vi "Launcher.vi"(9 "launcher_name":string, 10 "pid":u32) -> ()   [LabVIEW 2021, in "CIFLauncher.lvclass"]
uses:
  CIFLauncher.lvclass
  CIFLauncher.lvclass/CIFLauncher.ctl
  <vilib>/gRPC/LabVIEW gRPC Servicer/Servicer/Servicer.lvclass
  CIFUtilities/CIFLogs/CIFLogs.lvlib
  gRPC/CIF_Launcher_server/RPC Service/Launcher/Launcher.lvclass
  gRPC/CIF_Launcher_server/RPC Messages/cif_common_Empty.ctl
  gRPC/CIF_Launcher_server/CIF_Launcher_server.lvlib
  gRPC/CIF_Launcher_server/RPC Messages/cif_common_Version.ctl
  gRPC/CIF_Launcher_server/RPC Messages/cif_manager_PluginMetadata.ctl
  gRPC/CIF_Launcher_server/RPC Messages/cif_launcher_DiscoveredPlugin.ctl
  gRPC/CIF_Launcher_server/RPC Messages/cif_common_Status.ctl
  gRPC/CIF_Launcher_server/RPC Messages/cif_manager_LauncherType.ctl
  gRPC/CIF_Launcher_server/RPC Messages/cif_manager_LauncherInfo.ctl
  gRPC/CIF_Launcher_server/RPC Messages/cif_manager_LauncherStatus.ctl
  CIFUtilities/CIFConfigurationFile/typedef/Location Type.ctl
  CIFUtilities/CIFConfigurationFile/CIF Configuration File.lvlib
  <vilib>/Utility/LVLibp/NI_PackedLibraryUtility.lvlib
  CIFPluginManager/gRPC/CIF_Manager_Client_Wrapper/CIFManagerClientWrapper.lvlib
  gRPC/CIF_Launcher_server/RPC Messages/cif_launcher_DiscoveredPlugins.ctl
panel:
  out "error out":errorcluster
  in  "stop":bool
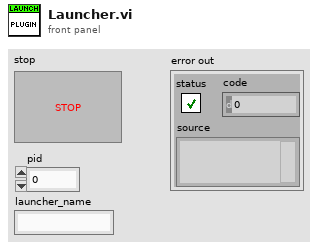
[diagram p1: front panel]
types:
  T1 = typedef "CIF_Launcher_server.lvlib/cif_launcher_DiscoveredPlugins.ctl" = cluster{"discovered_plugins":T2[], "status":T5}
  T2 = typedef "CIF_Launcher_server.lvlib/cif_launcher_DiscoveredPlugin.ctl" = cluster{"file_path":string, "file_name":string, "plugin_type":string, "plugin_version":T3, "plugin_metadata":T4}
  T3 = typedef "CIF_Launcher_server.lvlib/cif_common_Version.ctl" = cluster{"major":u32, "minor":u32, "fix":u32, "build":u32}
  T4 = typedef "CIF_Launcher_server.lvlib/cif_manager_PluginMetadata.ctl" = cluster{"description":string, "history":string, "author":string}
  T5 = typedef "CIF_Launcher_server.lvlib/cif_common_Status.ctl" = cluster{"code":i32, "message":string}
  T6 = typedef "CIF Configuration File.lvlib/Location Type.ctl" = enum16{"Config File", "Manager", "Protos", "Plugins", "UI Plugins", "Logs", "Orchestrations"}
  T7 = typedef "CIF_Launcher_server.lvlib/cif_common_Empty.ctl" = cluster{"void":string}
  T8 = typedef "CIF_Launcher_server.lvlib/cif_manager_LauncherStatus.ctl" = cluster{"launcher_info":T9, "grpc_port":i32, "pid":u32, "status":T5}
  T9 = typedef "CIF_Launcher_server.lvlib/cif_manager_LauncherInfo.ctl" = cluster{"launcher_type":T10, "launcher_name":string}
  T10 = typedef "CIF_Launcher_server.lvlib/cif_manager_LauncherType.ctl" = enum32{"LAUNCHERTYPE_UNKNOWN", "LAUNCHERTYPE_LABVIEW"}
  T11 = typedef "grpc-lvsupport-release.lvlib/grpcId.ctl" = u64
  T12 = typedef "CIF_Launcher_server.lvlib/cif_launcher_LaunchConfig.ctl" = cluster{"plugin_name":T13, "path":string}
  T13 = typedef "CIF_Launcher_server.lvlib/cif_manager_PluginName.ctl" = cluster{"plugin_name":string}
  T14 = typedef "CIFLauncher.lvclass/Loaded Plugin Map.ctl" = map{string, refnum<vi>}
  T15 = typedef "CIF_Launcher_server.lvlib/cif_launcher_DiscoverCommand.ctl" = cluster{"update_metadata":bool}
  T16 = typedef "trash_Discovered Plugin.ctl" = cluster{"Filename":string, "Plugin Type":string, "Qualified name":string, "Version":T17, "Plugin Metadata":T18}
  T17 = typedef "CIFCoreCommon.lvlib/Version.ctl" = cluster{"Major":i32, "Minor":i32, "Fix":i32, "Build":i32}
  T18 = typedef "trash_Plugin Metadata.ctl" = cluster{"Description":string, "History":string, "Author":string}
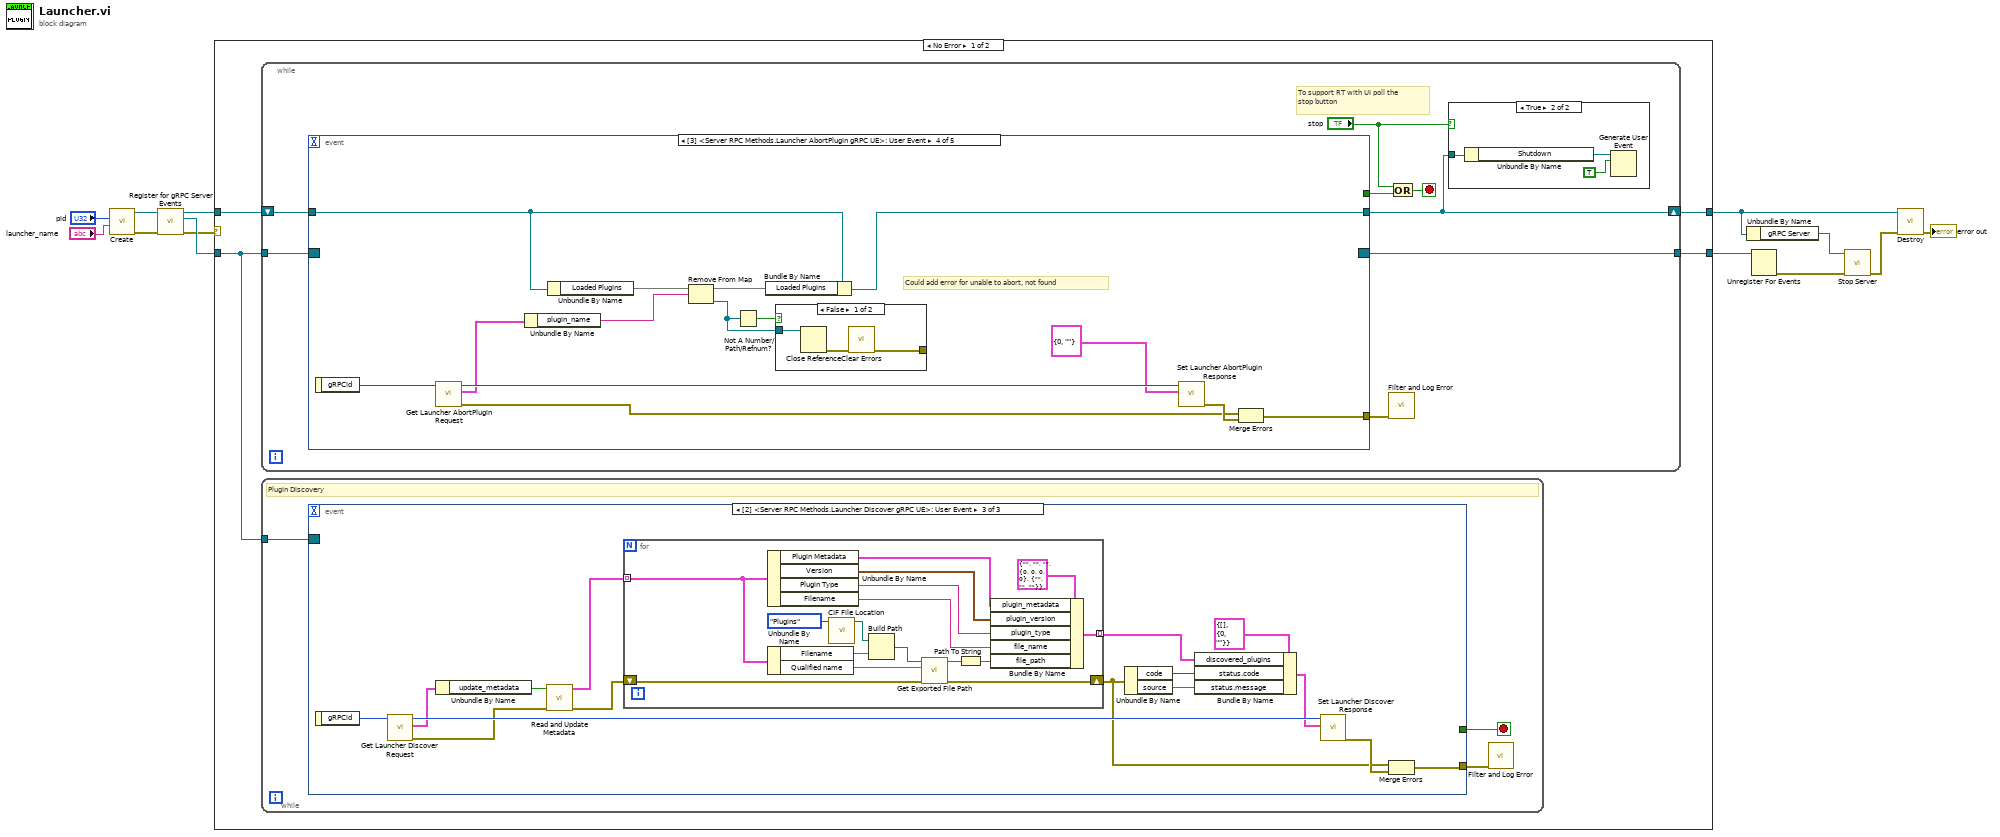
[diagram p0: block diagram]
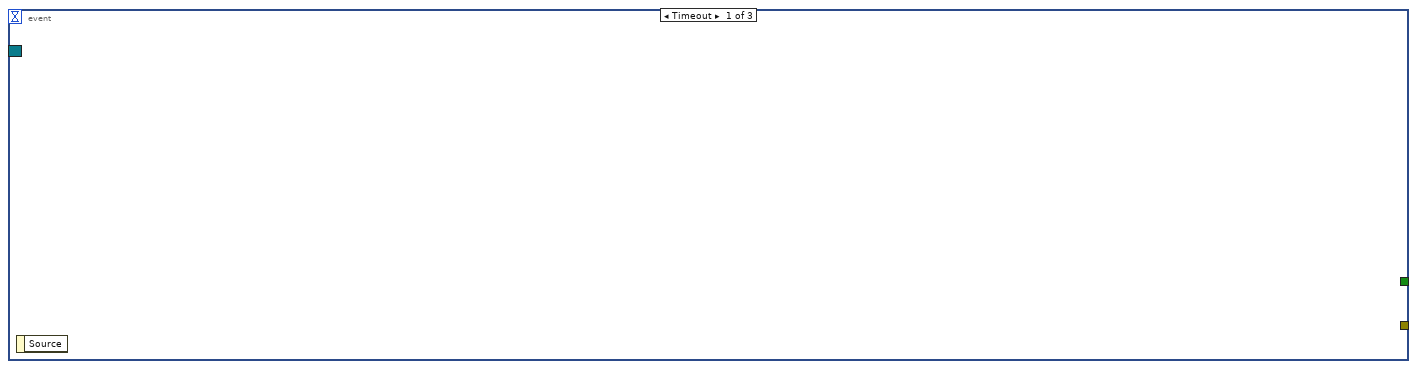
[diagram p2: hidden frame]
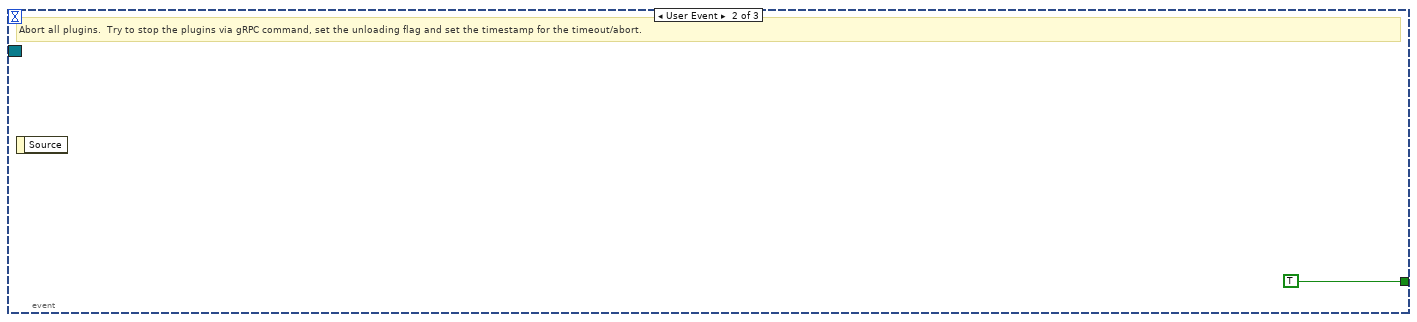
[diagram p3: hidden frame]
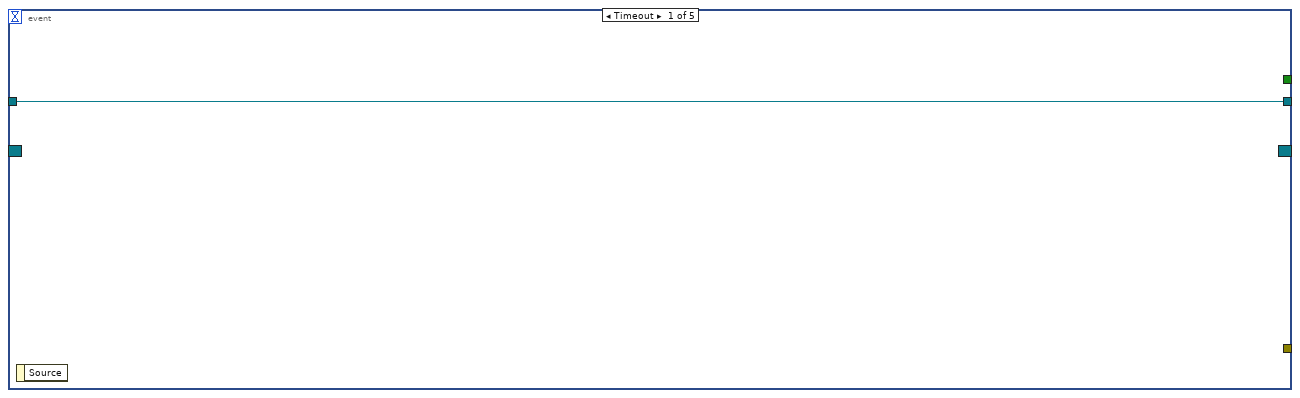
[diagram p5: hidden frame]
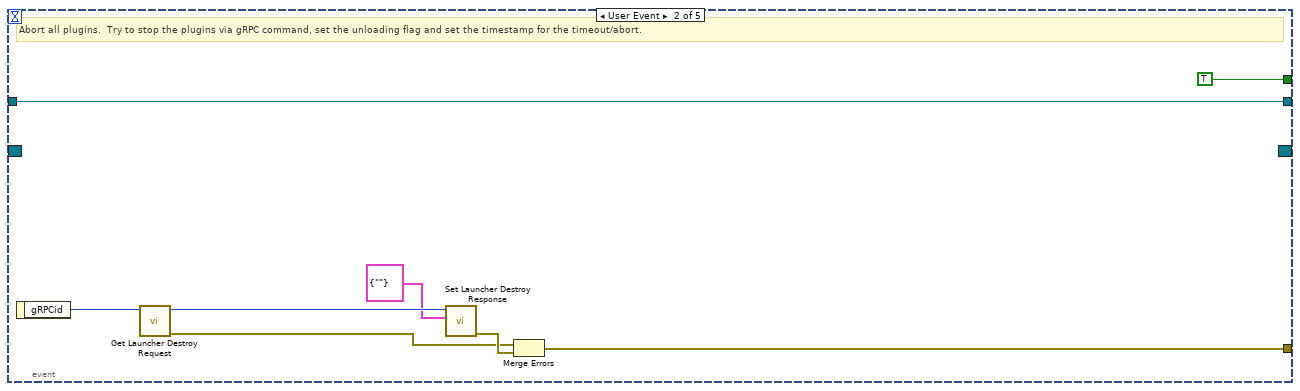
[diagram p6: hidden frame]
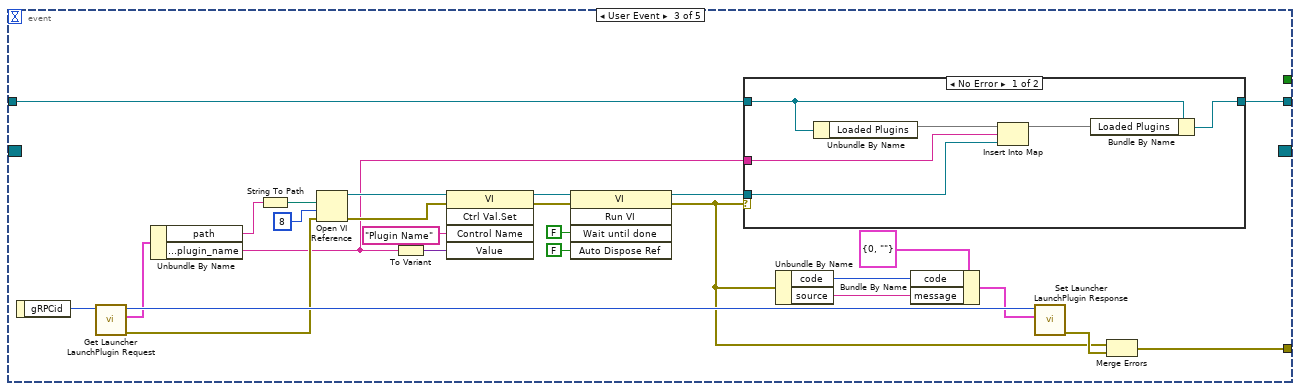
[diagram p7: hidden frame]
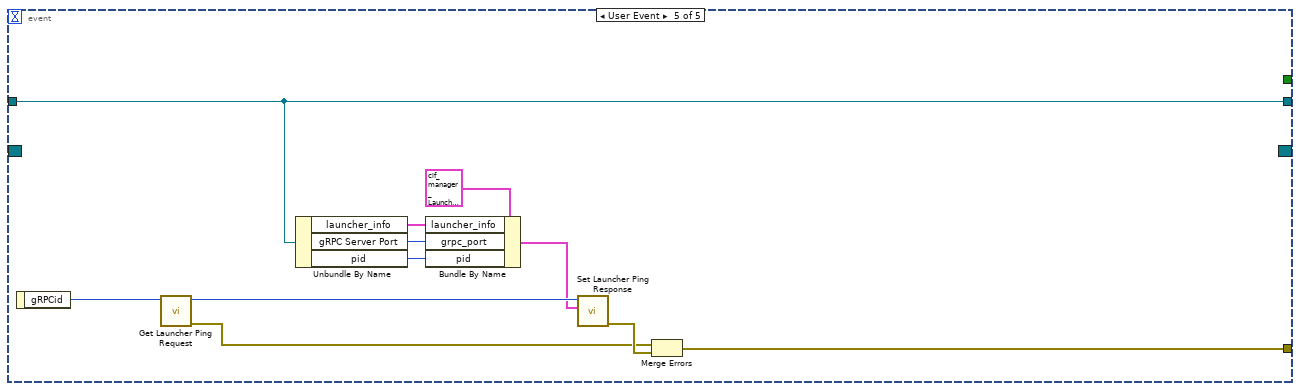
[diagram p10: hidden frame]
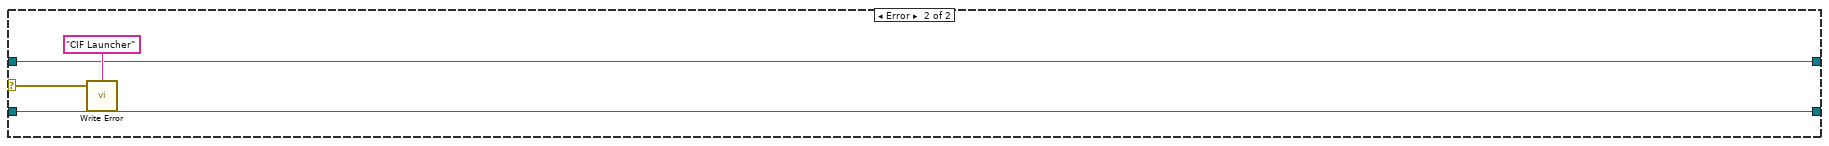
[diagram p11: hidden frame]
diagram:
  n1 = call "Create.vi"("launcher_name"="launcher_name", "pid"="pid") -> ("error out"=w5:errorcluster, "Plugin Manager out"=w6:refnum<class "CIFLauncher.lvclass">)  [unwired: 8 in]
  n2 = call "Register for gRPC Server Events.vi"("error in (no error)"=w5, "CIFLauncher in"=w6) -> ("error out"=w3:errorcluster, "Event Registration Refnum"=w4:refnum<event-registration>, "CIFLauncher out"=w7:refnum<class "CIFLauncher.lvclass">)  [unwired: 7 in]
  n3 = case shown="No Error" w3 {
    selector: w3 -> [_ w136]
    tunnel: [w17 w135] -> w8
    tunnel: [w16 w134] -> w9
    tunnel: w4 -> [w14 w134]
    tunnel: w7 -> [w15 w135]
    frame No Error {
      n4 = while {
        tunnel: w14 -> [w58]
        tunnel: [w59] -> w16
        shift-right: [w54] -> w17
        shift-left: w15 -> [w60]
        stop <- w56 stop-if-true
        # "To support RT with UI poll the stop button"
        n5 = event shown="[3] <Server RPC Methods.Launcher AbortPlugin gRPC UE>: User Event" {
          selector: w58 -> [_ _ _ _ _]
          dyn-events: [_ _ _ _ _] -> w59
          timeout: _ -> [_ _ _ _ _]
          tunnel: w60 -> [w64 w70 w81 w111 w125]
          tunnel: [w64 w70 w78 w106 w125] -> w54
          tunnel: [_ w72 w83 w114 w130] -> w53
          tunnel: [_ TRUE _ _ _] -> w57
          event Timeout {
            n6 = event-data() -> ()  [unwired: 1 in, 1 out]
          }
          event User Event {
            # "Abort all plugins.  Try to stop the plugins via gRPC command, set the unloading flag and set the timestamp for the timeout/abort."
            n7 = event-data() -> ("gRPCid"=w69:T11)  [unwired: 1 in]
            n8 = call "Get Launcher Destroy Request.vi"("gRPCid"=w69) -> ("error out"=w65:errorcluster, "gRPCid out"=w68:T11)  [unwired: 8 in, 1 out]
            n9 = call "Set Launcher Destroy Response.vi"("Message Data"=T7 {"void"=""}, "gRPCid in"=w68) -> ("error out"=w66:errorcluster)  [unwired: 9 in]
            n10 = Merge Errors(w65, w66) -> (w72:errorcluster)
          }
          event User Event {
            n11 = event-data() -> ("gRPCid"=w98:T11)  [unwired: 1 in]
            n12 = call "Get Launcher LaunchPlugin Request.vi"("gRPCid"=w98) -> ("error out"=w85:errorcluster, "Message Data"=w96:T12, "gRPCid out"=w97:T11)  [unwired: 8 in]
            n13 = Unbundle By Name(w96) -> ("path"=w87:string, "plugin_name.plugin_name"=w80:string)
            n14 = String To Path(string=w87) -> (path=w86:path)
            n15 = Open VI Reference(vi path=w86, options=8, error in (no error)=w85) -> (vi reference=w90:refnum<vi>, error out=w93:errorcluster)  [unwired: 3 in]
            n16 = To Variant(anything=w80) -> (Variant=w88:variant)
            n17 = invoke class="VI" method="Ctrl Val.Set"(reference=w90, error in=w93, "Control Name"="Plugin Name", "Value"=w88) -> (reference out=w92:refnum<vi>, error out=w91:errorcluster)  [unwired: 1 in, 3 out]
            n18 = invoke class="VI" method="Run VI"(reference=w92, error in=w91, "Wait until done"=FALSE ("Wait Until Done"), "Auto Dispose Ref"=FALSE ("Auto Dispose Reference")) -> (reference out=w79:refnum<vi>, error out=w76:errorcluster)  [unwired: 1 in, 3 out]
            n19 = case shown="No Error" w76 {
              tunnel: w81 -> [w104 w105]
              tunnel: w80 -> [w102 _]
              tunnel: w79 -> [w101 _]
              tunnel: [w99 w105] -> w78
              frame No Error {
                n20 = Unbundle By Name(w104) -> ("Loaded Plugins"=w103:T14)
                n21 = Insert Into Map(map in=w103, key=w102, value=w101) -> (map out=w100:T14)  [unwired: 2 out]
                n22 = Bundle By Name(cluster=w104, "Loaded Plugins"=w100) -> (w99:refnum<class "CIFLauncher.lvclass">)
              }
              frame Error {
              }
            }
            n23 = Unbundle By Name(w76) -> ("code"=w74:i32, "source"=w75:string)
            n24 = Bundle By Name(cluster=T5 {"code"=0, "message"=""} ("Message Data"), "code"=w74, "message"=w75) -> (w73:T5)
            n25 = call "Set Launcher LaunchPlugin Response.vi"("Message Data"=w73, "gRPCid in"=w97) -> ("error out"=w84:errorcluster)  [unwired: 9 in]
            n26 = Merge Errors(w76, w84) -> (w83:errorcluster)
          }
          event User Event {
            # "Could add error for unable to abort, not found"
            n27 = event-data() -> ("gRPCid"=w119:T11)  [unwired: 1 in]
            n28 = call "Get Launcher AbortPlugin Request.vi"("gRPCid"=w119) -> ("error out"=w113:errorcluster, "Message Data"=w117:T13, "gRPCid out"=w118:T11)  [unwired: 8 in]
            n29 = Unbundle By Name(w117) -> ("plugin_name"=w108:string)
            n30 = Unbundle By Name(w111) -> ("Loaded Plugins"=w109:T14)
            n31 = Remove From Map(10:w108, 11:w109) -> (1:w107:refnum<vi>, 3:w110:T14)  [unwired: 1 out]
            n32 = Not A Number/Path/Refnum?(number/path/refnum=w107) -> (NaN/Path/Refnum?=w112:bool)
            n33 = Bundle By Name(cluster=w111, "Loaded Plugins"=w110) -> (w106:refnum<class "CIFLauncher.lvclass">)
            n34 = case shown="False" w112 {
              tunnel: w107 -> [w122 _]
              tunnel: [w120 _] -> _
              frame False {
                n35 = Close Reference(reference=w122) -> (error out=w121:errorcluster)  [unwired: 1 in]
                n36 = call <vilib>:"Clear Errors.vi"("error in (no error)"=w121) -> ("error out"=w120:errorcluster)  [unwired: 5 in, 1 out]
              }
              frame True {
              }
            }
            n37 = call "Set Launcher AbortPlugin Response.vi"("Message Data"=T5 {"code"=0, "message"=""}, "gRPCid in"=w118) -> ("error out"=w115:errorcluster)  [unwired: 9 in]
            n38 = Merge Errors(w113, w115) -> (w114:errorcluster)
          }
          event User Event {
            n39 = event-data() -> ("gRPCid"=w133:T11)  [unwired: 1 in]
            n40 = call "Get Launcher Ping Request.vi"("gRPCid"=w133) -> ("error out"=w129:errorcluster, "gRPCid out"=w132:T11)  [unwired: 8 in, 1 out]
            n41 = Unbundle By Name(w125) -> ("launcher_info"=w128:T9, "gRPC Server Port"=w127:i32, "pid"=w126:u32)
            n42 = Bundle By Name(cluster=T8 {"launcher_info"={"launcher_type"=enum."LAUNCHERTYPE_UNKNOWN", "launcher_name"=""}, "grpc_port"=0, "pid"=0, "status"={"code"=0, "message"=""}} ("Message Data"), "launcher_info"=w128, "grpc_port"=w127, "pid"=w126) -> (w123:T8)
            n43 = call "Set Launcher Ping Response.vi"("Message Data"=w123, "gRPCid in"=w132) -> ("error out"=w131:errorcluster)  [unwired: 9 in]
            n44 = Merge Errors(w129, w131) -> (w130:errorcluster)
          }
        }
        n45 = call "Filter and Log Error.vi"("error In"=w53) -> ()  [unwired: 11 in]
        n46 = Compound Arithmetic op=OR("stop", w57) -> (w56:bool)
        n47 = case shown="True" "stop" {
          tunnel: w54 -> [_ w61]
          frame False {
          }
          frame True {
            n48 = Unbundle By Name(w61) -> ("Shutdown"=w62:refnum<user-event>)
            n49 = Generate User Event(user event=w62, event data cluster=TRUE ("event data")) -> ()  [unwired: 2 in, 2 out]
          }
        }
      }
      n50 = while {
        tunnel: w14 -> [w20]
        stop <- w18 stop-if-true
        # "Plugin Discovery"
        n51 = event shown="[2] <Server RPC Methods.Launcher Discover gRPC UE>: User Event" {
          selector: w20 -> [_ _ _]
          dyn-events: _ -> [_ _ _]
          timeout: _ -> [_ _ _]
          tunnel: [_ _ w30] -> w19
          tunnel: [_ TRUE _] -> w18
          event Timeout {
            n52 = event-data() -> ()  [unwired: 1 in, 1 out]
          }
          event User Event {
            # "Abort all plugins.  Try to stop the plugins via gRPC command, set the unloading flag and set the timestamp for the timeout/abort."
            n53 = event-data() -> ()  [unwired: 1 in, 1 out]
          }
          event User Event {
            n54 = event-data() -> ("gRPCid"=w36:T11)  [unwired: 1 in]
            n55 = call "Get Launcher Discover Request.vi"("gRPCid"=w36) -> ("error out"=w32:errorcluster, "Message Data"=w34:T15, "gRPCid out"=w35:T11)  [unwired: 8 in]
            n56 = Unbundle By Name(w34) -> ("update_metadata"=w33:bool)
            n57 = call "Read and Update Metadata.vi"("error in (no error)"=w32, "Update Metadata"=w33) -> ("error out"=w28:errorcluster, "Plugin Info"=w29:T16[])  [unwired: 8 in]
            n58 = for {
              tunnel: w29 -> [w50] mode=indexing
              shift-right: [w51] -> w22
              shift-left: w28 -> [w52]
              tunnel: [w42] -> w25 mode=indexing
              n59 = Unbundle By Name(w50) -> ("Plugin Metadata"=w43:T18, "Version"=w44:T17, "Plugin Type"=w45:string, "Filename"=w46:string)
              n60 = Unbundle By Name(w50) -> ("Filename"=w40:string, "Qualified name"=w39:string)
              n61 = call "CIF File Location.vi"("LocationType"=Location_Type."Plugins") -> ("Location"=w37:path)  [unwired: 10 in]
              n62 = Build Path(base path=w37, name or relative path=w40) -> (appended path=w41:path)
              n63 = call <vilib>:"Get Exported File Path.vi"("error in (no error)"=w52, "qualified name"=w39, "packed library path"=w41) -> ("error out"=w51:errorcluster, "path"=w48:path)  [unwired: 7 in]
              n64 = Path To String(path=w48) -> (string=w47:string)
              n65 = Bundle By Name(cluster=T2 {"file_path"="", "file_name"="", "plugin_type"="", "plugin_version"={"major"=0, "minor"=0, "fix"=0, "build"=0}, "plugin_metadata"={"description"="", "history"="", "author"=""}} ("cif_launcher_DiscoveredPlugin"), "plugin_metadata"=w43, "plugin_version"=w44, "plugin_type"=w45, "file_name"=w46, "file_path"=w47) -> (w42:T2)
            }
            n66 = Unbundle By Name(w22) -> ("code"=w27:i32, "source"=w24:string)
            n67 = Bundle By Name(cluster=T1 {"discovered_plugins"=[], "status"={"code"=0, "message"=""}} ("Message Data"), "discovered_plugins"=w25, "status.code"=w27, "status.message"=w24) -> (w23:T1)
            n68 = call "Set Launcher Discover Response.vi"("Message Data"=w23, "gRPCid in"=w35) -> ("error out"=w31:errorcluster)  [unwired: 9 in]
            n69 = Merge Errors(w22, w31) -> (w30:errorcluster)
          }
        }
        n70 = call "Filter and Log Error.vi"("error In"=w19) -> ()  [unwired: 11 in]
      }
    }
    frame Error {
      n71 = call "Write Error.vi"("error in (no error)"=w136, "Plugin Name"="CIF Launcher") -> ()  [unwired: 2 in, 1 out]
    }
  }
  n72 = Unbundle By Name(w8) -> ("gRPC Server"=w12:refnum<class "Servicer.lvclass">)
  n73 = Unregister For Events(event registration refnum=w9) -> (error out=w13:errorcluster)  [unwired: 1 in]
  n74 = call <vilib>:"Stop Server.vi"("error in"=w13, "gRPC Server in"=w12) -> ("error out"=w11:errorcluster)  [unwired: 9 in]
  n75 = call "Destroy.vi"("error in (no error)"=w11, "Plugin Manager in"=w8) -> ("error out"=→"error out":errorcluster)  [unwired: 8 in, 1 out]
